vi "GLOBAL_VernierCals_Dig1.vi"(9 "Digitizer1 IN":T1={"MAXVER_0"=13030, "MINVER_0"=11830, "MAXVER_1"=12945, "MINVER_1"=11712, "MAXVER_2"=13022, "MINVER_2"=11775, "MAXVER_3"=12900, "MINVER_3"=11779}, 10 "State":enum16{"Initialise", "Write", "Read"}(ring)) -> (1 "Digitizer1 OUT":T1={"MAXVER_0"=13030, "MINVER_0"=11830, "MAXVER_1"=12945, "MINVER_1"=11712, "MAXVER_2"=13022, "MINVER_2"=11775, "MAXVER_3"=12900, "MINVER_3"=11779})   [LabVIEW 2014]
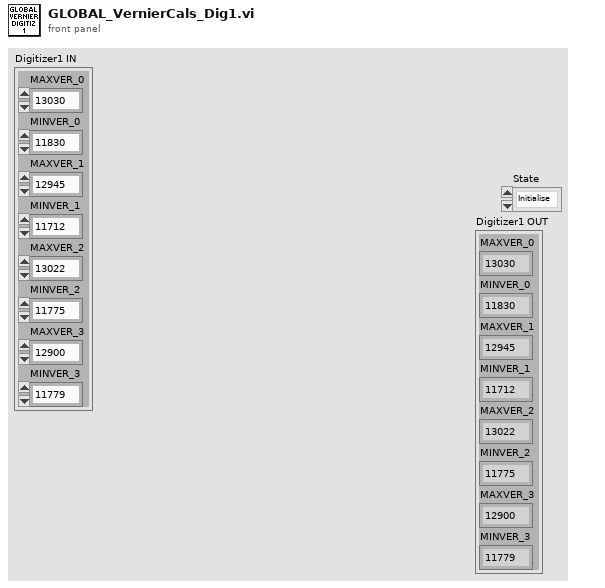
[diagram p1: front panel]
types:
  T1 = cluster{"MAXVER_0":u16, "MINVER_0":u16, "MAXVER_1":u16, "MINVER_1":u16, "MAXVER_2":u16, "MINVER_2":u16, "MAXVER_3":u16, "MINVER_3":u16}
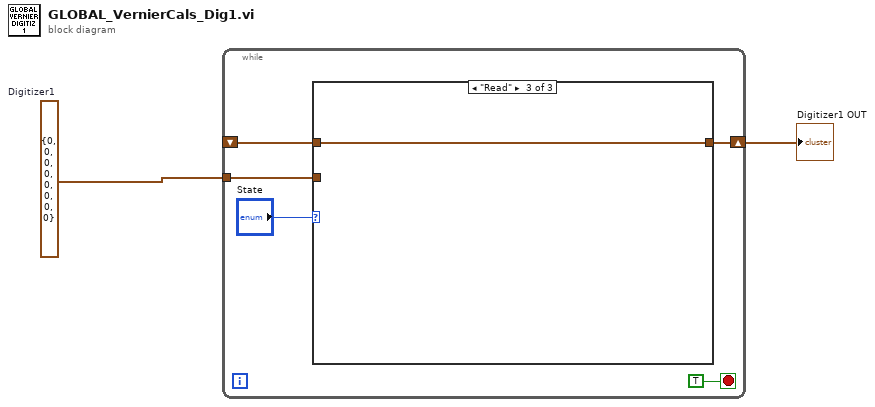
[diagram p0: block diagram]
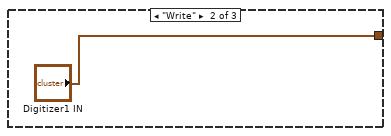
[diagram p3: hidden frame]
diagram:
  w2 = T1 {"MAXVER_0"=0, "MINVER_0"=0, "MAXVER_1"=0, "MINVER_1"=0, "MAXVER_2"=0, "MINVER_2"=0, "MAXVER_3"=0, "MINVER_3"=0}  # Digitizer1
  n1 = while {
    tunnel: w2 -> [w6]
    shift-right: [w5] -> w1
    shift-left: _ -> [w4]
    stop <- TRUE stop-if-true
    n2 = case shown="\"Read\"" "State" {
      tunnel: w6 -> [w8 _ _]
      tunnel: [w8 "Digitizer1 IN" w10] -> w5
      tunnel: w4 -> [_ _ w10]
      frame "Initialise", Default {
      }
      frame "Write" {
      }
      frame "Read" {
      }
    }
  }
  "Digitizer1 OUT" <- w1
